vi "Mediaplayer play LOOP.vi"(8 "error in (no error)":errorcluster, 10 "playState in":i32, 11 "Automation Refnum in":refnum<k7>) -> (0 "error out":errorcluster, 3 "playState out":i32)   [LabVIEW 2010]
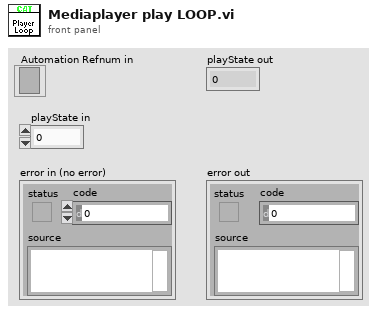
[diagram p1: front panel]
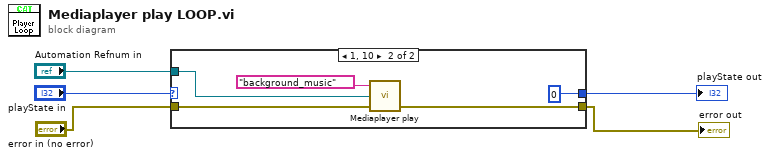
[diagram p0: block diagram]
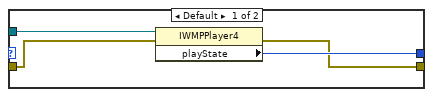
[diagram p2: hidden frame]
diagram:
  n1 = case shown="1, 10" "playState in" {
    tunnel: "Automation Refnum in" -> [w9 w13]
    tunnel: [w8 0 ("playState")] -> w1
    tunnel: "error in (no error)" -> [w7 w11]
    tunnel: [w6 w10] -> w3
    frame Default {
      n2 = property class="IWMPPlayer4"(reference=w9, error in=w7) -> (error out=w6:errorcluster, "playState"=w8:i32)  [unwired: 1 out]
    }
    frame 1, 10 {
      n3 = call "Mediaplayer play.vi"("music"="background_music", "MediaPlayer"=w13, "error in"=w11) -> ("error out"=w10:errorcluster)  [unwired: 4 in]
    }
  }
  "error out" <- w3
  "playState out" <- w1
